vi "Apply_New_Window_Center.vi"(9 "ResetTrig":bool, 10 "User Trig":T2, 11 "FeedbackTrig":T1) -> (2 "AllWindows out":T2)   [LabVIEW 2021]
doc: "Use this VI to update the window center.\nWhen we trigger (on the high side or the low side of the trigger window), use the triggering signal value as the new window center.\nLuke 11-18-2022"
uses:
  Host/Clusts/AllWindowsClust.ctl
  Host/Clusts/ChannelWindowClust.ctl
  Controls/Clust/Update_Trigger_Center.ctl
panel:
  in  "Chan# (only Channel 0 works now)":i16
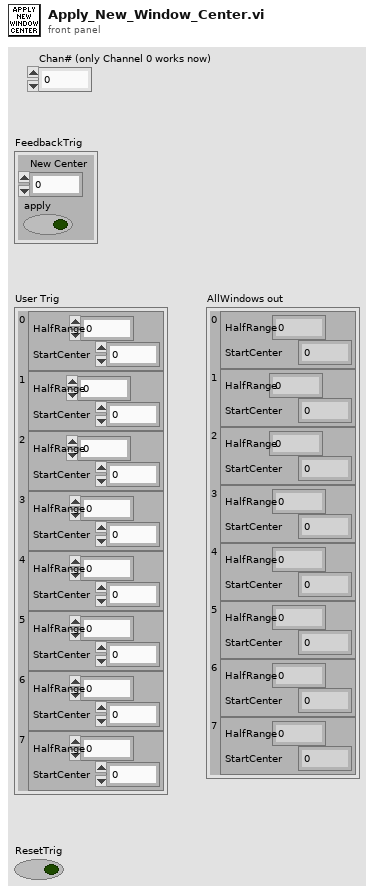
[diagram p1: front panel]
types:
  T1 = typedef "Update_Trigger_Center.ctl" = cluster{"New Center":fxp<+/-,18,5>, "apply":bool}
  T2 = typedef "AllWindowsClust.ctl" = cluster{"0":T3, "1":T3, "2":T3, "3":T3, "4":T3, "5":T3, "6":T3, "7":T3}
  T3 = typedef "ChannelWindowClust.ctl" = cluster{"HalfRange":fxp<+/-,18,5>, "StartCenter":fxp<+/-,18,5>}
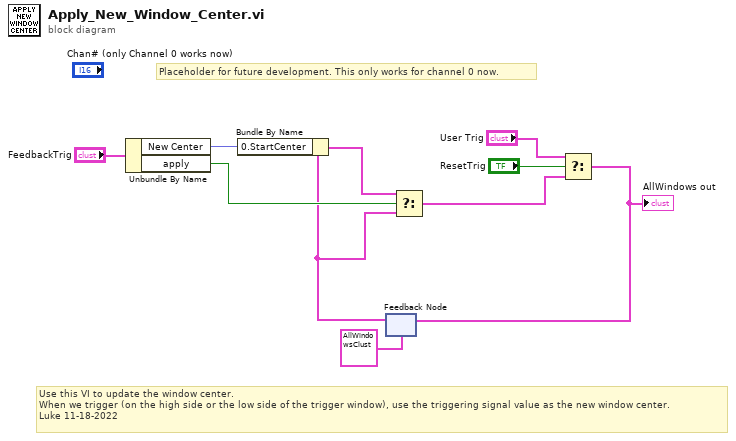
[diagram p0: block diagram]
diagram:
  # "Placeholder for future development. This only works for channel 0 now."
  # "Use this VI to update the window center.\nWhen we trigger (on the high side or the low side of the trigger window), use the triggering signal value as the new window center.\nLuke 11-18-2022"
  n1 = Unbundle By Name("FeedbackTrig") -> ("New Center"=w8:fxp<+/-,18,5>, "apply"=w7:bool)
  n2 = feedback #1(T2 {"0"={"HalfRange"=0.0, "StartCenter"=0.0}, "1"={"HalfRange"=0.0, "StartCenter"=0.0}, "2"={"HalfRange"=0.0, "StartCenter"=0.0}, "3"={"HalfRange"=0.0, "StartCenter"=0.0}, "4"={"HalfRange"=0.0, "StartCenter"=0.0}, "5"={"HalfRange"=0.0, "StartCenter"=0.0}, "6"={"HalfRange"=0.0, "StartCenter"=0.0}, "7"={"HalfRange"=0.0, "StartCenter"=0.0}} ("User Trig")) -> (w2:T2)
  n3 = Bundle By Name(cluster=w2, "0.StartCenter"=w8) -> (w10:T2)
  n4 = Select(t=w10, s=w7, f=w2) -> (s? t:f=w3:T2)
  n5 = Select(t="User Trig", s="ResetTrig", f=w3) -> (s? t:f=w1:T2)
  "AllWindows out" <- w1
  n6 = feedback-in #1(w1) -> ()
